vi "ExParamInfo.vi"() -> ()   [LabVIEW 2010]
panel:
  in  "Param ID":u32
  out "Description":string
  out "Number of Enums":u32
  out "Bit Used Flag":u32 format="%.0x"
  out "Access Type":u32
  out "Data Type":u32
  out "Increment":dbl format="%.2f"
  out "Max Value":dbl format="%.2f"
  out "Min Value":dbl format="%.2f"
  out "Default Value":dbl format="%.2f"
  out "Current Value":dbl format="%.2f"
  out "Avail Flag":u8
  out "Param ID":u32
  out "error out":errorcluster
  in  "error in (no error)":errorcluster
  # "ExParamInfo:\nThis example shows how to use the\nParam ID Get Functions. Enter parameter\nID below and to the right if it exists you \nwill see the results."
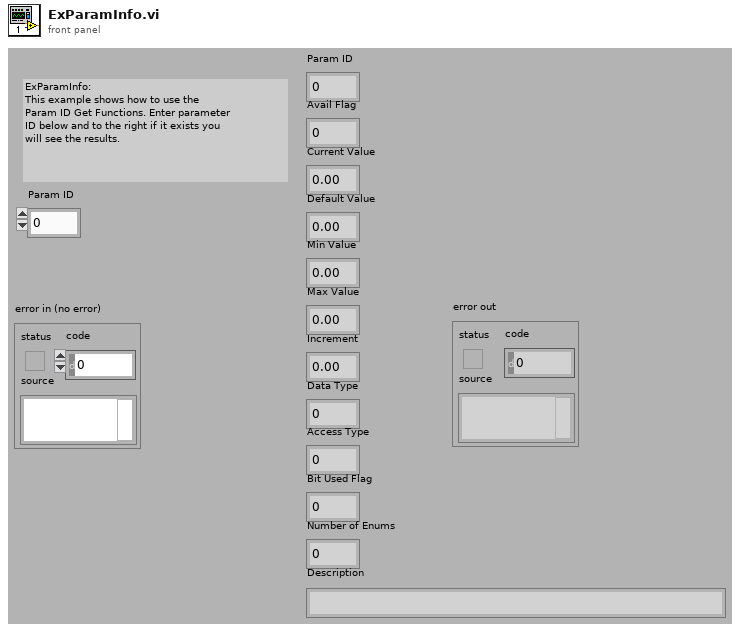
[diagram p1: front panel]
types:
  T1 = cluster{"Param ID":u32, "Avail Flag":u8, "Current Value":dbl, "Default Value":dbl, "Min Value":dbl, "Max Value":dbl, "Increment":dbl, "Data Type":u32, "Access Type":u32, "Bit Used Flag":u32, "Number of Enums":u32, "Description":string}
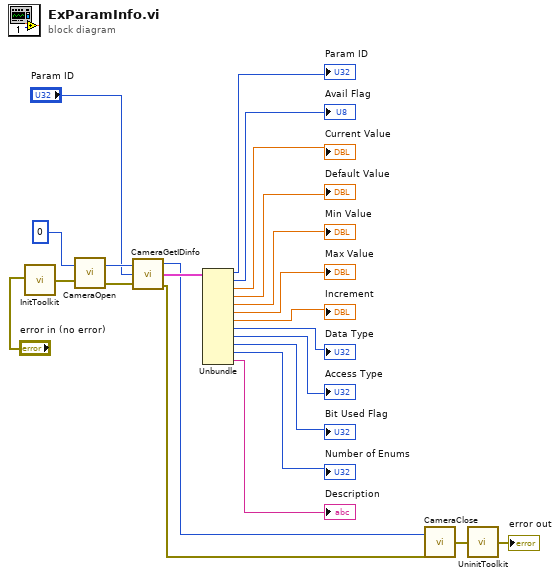
[diagram p0: block diagram]
diagram:
  n1 = call <userlib>:"InitToolkit.vi"("error in"="error in (no error)") -> ("error out"=w23:errorcluster)
  n2 = call <userlib>:"CameraOpen.vi"("error in"=w23, "Camera Device ID"=0) -> ("error out"=w17:errorcluster, "Camera Handle"=w18:u32)
  n3 = call <userlib>:"CameraGetIDinfo.vi"("error in"=w17, "Param ID"="Param ID", "Camera handle"=w18) -> ("error out"=w2:errorcluster, "Param ID Information"=w19:T1, "Camera handle"=w1:u32)
  n4 = Unbundle(w19) -> ("Param ID"=→"Param ID":u32, "Avail Flag"=→"Avail Flag":u8, "Current Value"=→"Current Value":dbl, "Default Value"=→"Default Value":dbl, "Min Value"=→"Min Value":dbl, "Max Value"=→"Max Value":dbl, "Increment"=→"Increment":dbl, "Data Type"=→"Data Type":u32, "Access Type"=→"Access Type":u32, "Bit Used Flag"=→"Bit Used Flag":u32, "Number of Enums"=→"Number of Enums":u32, "Description"=→"Description":string)
  n5 = call <userlib>:"CameraClose.vi"("error in"=w2, "Camera Handle"=w1) -> ("error out"=w4:errorcluster)
  n6 = call <userlib>:"UninitToolkit.vi"("error in"=w4) -> ("error out"=→"error out":errorcluster)
